vi "Fetch Sensor Data.vi"(8 "error in (no error)":errorcluster, 9 "SensorID":i32, 11 "Database":refnum<queue>) -> (0 "error out":errorcluster, 2 "Data Valid?":bool, 3 "Sensor CoreData Cluster":T1)   [LabVIEW 2026, in "Settings.lvlib"]
uses:
  support/Architecture/Message Queue/Message Cluster.ctl
  controls/Messaging Payloads/Sensor FetchResponse.ctl
  support/Architecture/Message Queue/Enqueue Message (Single).vi
  Settings/Settings.lvlib
  controls/Messaging Payloads/Sensor CoreData Cluster.ctl
  controls/UI/Units Enum.ctl
  controls/UI/Signal Enum.ctl
  support/Architecture/Message Queue/Message Queue.lvlib
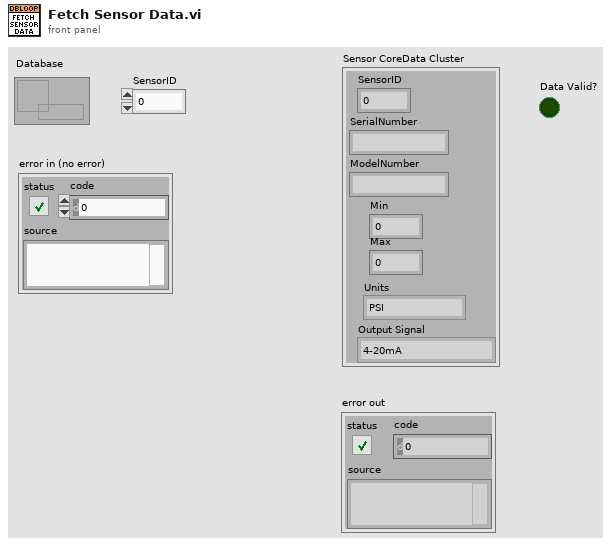
[diagram p1: front panel]
types:
  T1 = typedef "Settings.lvlib/Sensor CoreData Cluster.ctl" = cluster{"SensorID":i32, "SerialNumber":string, "ModelNumber":string, "Min":dbl, "Max":dbl, "Units":T2, "Output Signal":T3}
  T2 = typedef "Units Enum.ctl" = enum16{"PSI", "Deg C", "kPa", "GPM"}
  T3 = typedef "Signal Enum.ctl" = enum16{"4-20mA", "0-10V", "Thermocouple Type K"}
  T4 = typedef "Sensor FetchResponse.ctl" = cluster{"Notifier":refnum<notifier>, "Sensor ID":i32}
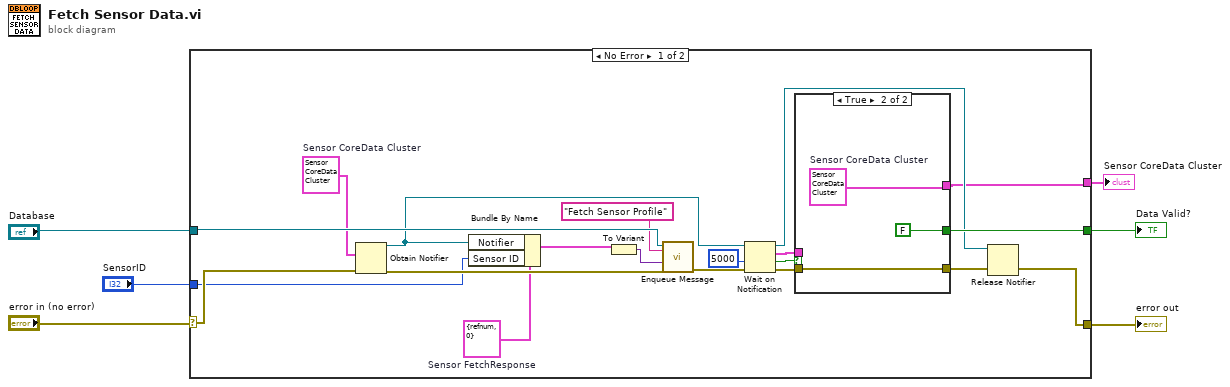
[diagram p0: block diagram]
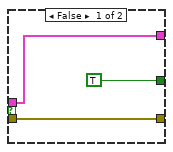
[diagram p2: hidden frame]
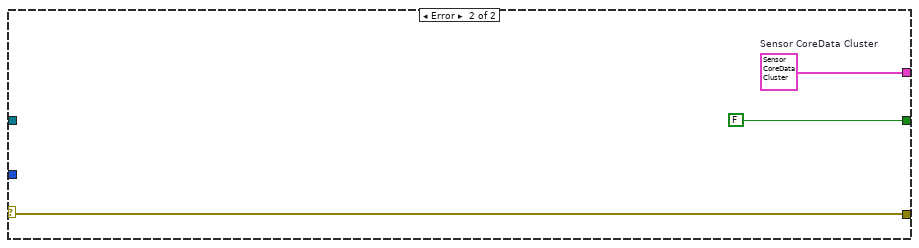
[diagram p3: hidden frame]
diagram:
  n1 = case shown="No Error" "error in (no error)" {
    selector: "error in (no error)" -> [w23 w35]
    tunnel: [w26 w35] -> w6
    tunnel: "Database" -> [w25 _]
    tunnel: [w24 FALSE] -> w3
    tunnel: "SensorID" -> [w8 _]
    tunnel: [w7 w33] -> w1
    frame No Error {
      w9 = T1 {"SensorID"=0, "SerialNumber"="", "ModelNumber"="", "Min"=0.0, "Max"=0.0, "Units"=enum."PSI", "Output Signal"=enum."4-20mA"}  # Sensor CoreData Cluster
      w17 = T4 {"Notifier"=refnum, "Sensor ID"=0}  # Sensor FetchResponse
      n2 = Obtain Notifier(notification data type=w9, error in (no error)=w23) -> (notifier out=w10:refnum<notifier>, error out=w22:errorcluster)  [unwired: 2 in, 1 out]
      n3 = Bundle By Name(cluster=w17, "Notifier"=w10, "Sensor ID"=w8) -> (w20:T4)
      n4 = To Variant(anything=w20) -> (Variant=w19:variant)
      n5 = call-poly "Enqueue Message.vi"("error in (no error)"=w22, "Message Data"=w19, "Message"="Fetch Sensor Profile", "Message Queue"=w25) -> ("error out"=w21:errorcluster)  [unwired: 6 in, 1 out]
      n6 = Wait on Notification(notifier=w10, timeout in ms (-1)=5000, error in (no error)=w21) -> (notifier out=w14:refnum<notifier>, notification=w11:T1, timed out?=w15:bool, error out=w13:errorcluster)  [unwired: 1 in]
      n7 = case shown="True" w15 {
        tunnel: w13 -> [w29 w32]
        tunnel: [w29 w32] -> w12
        tunnel: w11 -> [w27 _]
        tunnel: [w27 w30] -> w7
        tunnel: [TRUE FALSE] -> w24
        frame False {
        }
        frame True {
          w30 = T1 {"SensorID"=0, "SerialNumber"="", "ModelNumber"="", "Min"=0.0, "Max"=0.0, "Units"=enum."PSI", "Output Signal"=enum."4-20mA"}  # Sensor CoreData Cluster
        }
      }
      n8 = Release Notifier(notifier=w14, error in (no error)=w12) -> (error out=w26:errorcluster)  [unwired: 1 in, 2 out]
    }
    frame Error {
      w33 = T1 {"SensorID"=0, "SerialNumber"="", "ModelNumber"="", "Min"=0.0, "Max"=0.0, "Units"=enum."PSI", "Output Signal"=enum."4-20mA"}  # Sensor CoreData Cluster
    }
  }
  "error out" <- w6
  "Data Valid?" <- w3
  "Sensor CoreData Cluster" <- w1
